vi "Calibrate.vi"() -> ()   [LabVIEW 2017]
panel:
  in  "Make New Calibration Setup":bool
  in  "Quit Calibration":bool
  in  "Load R.M.":bool
  in  "Load n":bool
  in  "Load S.F.":bool
  in  "Load P.M.":bool
  in  "Load Axial":bool
  in  "Load N.B.":bool
  out "Calibration Complete":bool
  out "Rolling Moment":bool
  out "n":bool
  out "S.F.":bool
  out "P.M.":bool
  out "Axial":bool
  out "Normal Beam":bool
  out "Current Calibration File Path":path
  in  "Load":bool
  in  "Use Old Calibration File Path":path
  # "Calibration Status"
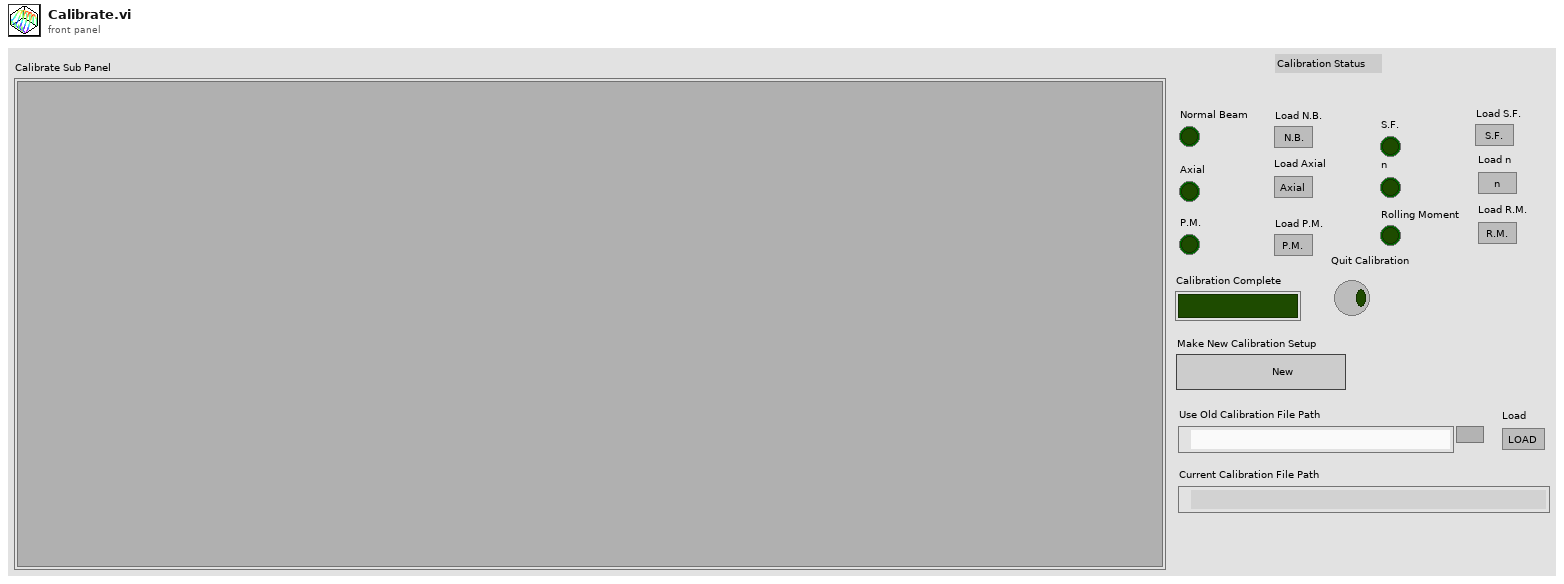
[diagram p1: front panel]
types:
  T1 = enum16{"open", "replace", "create", "open or create", "replace or create", "replace or create with confirmation"}
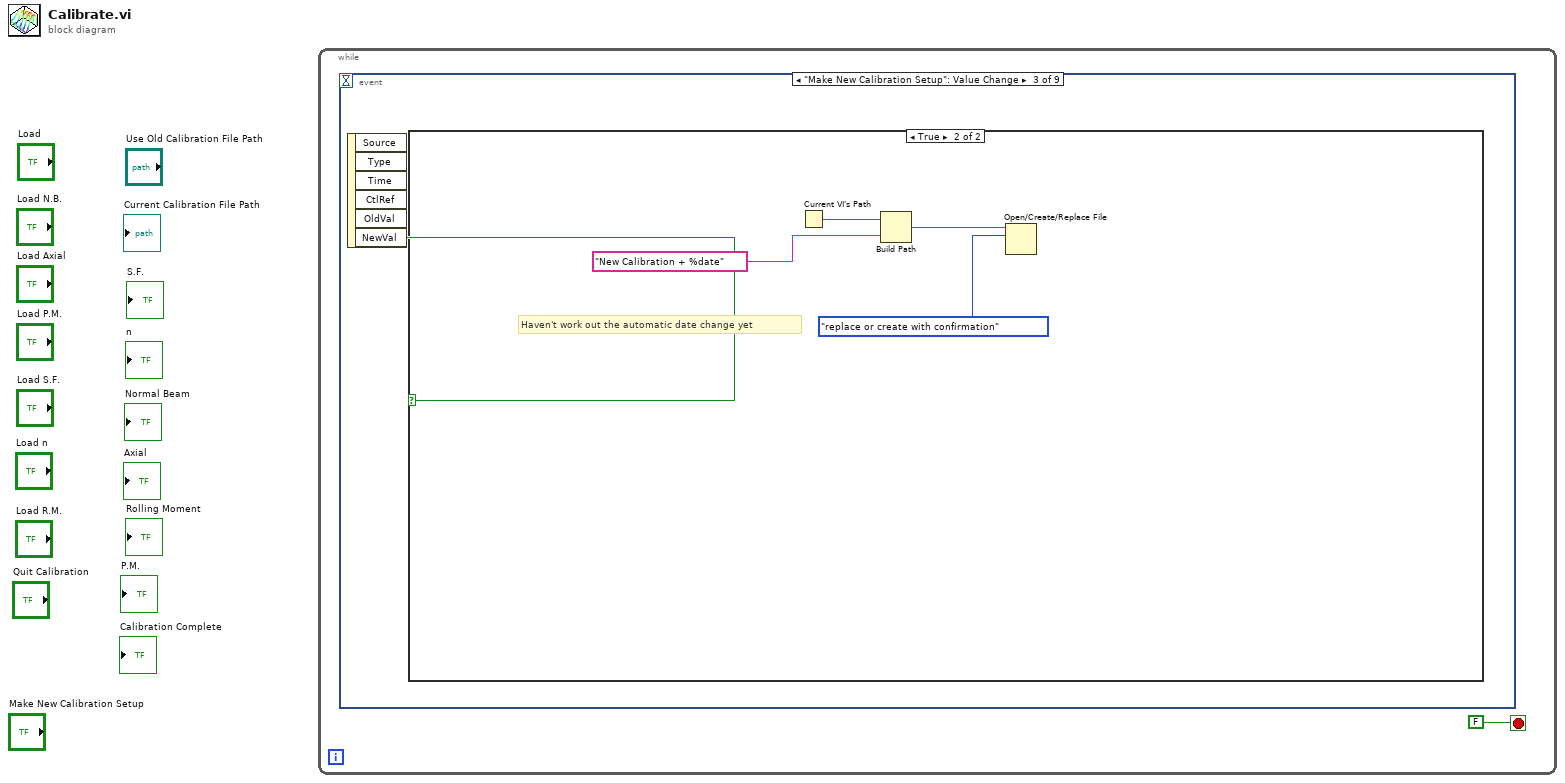
[diagram p0: block diagram]
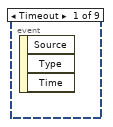
[diagram p2: hidden frame]
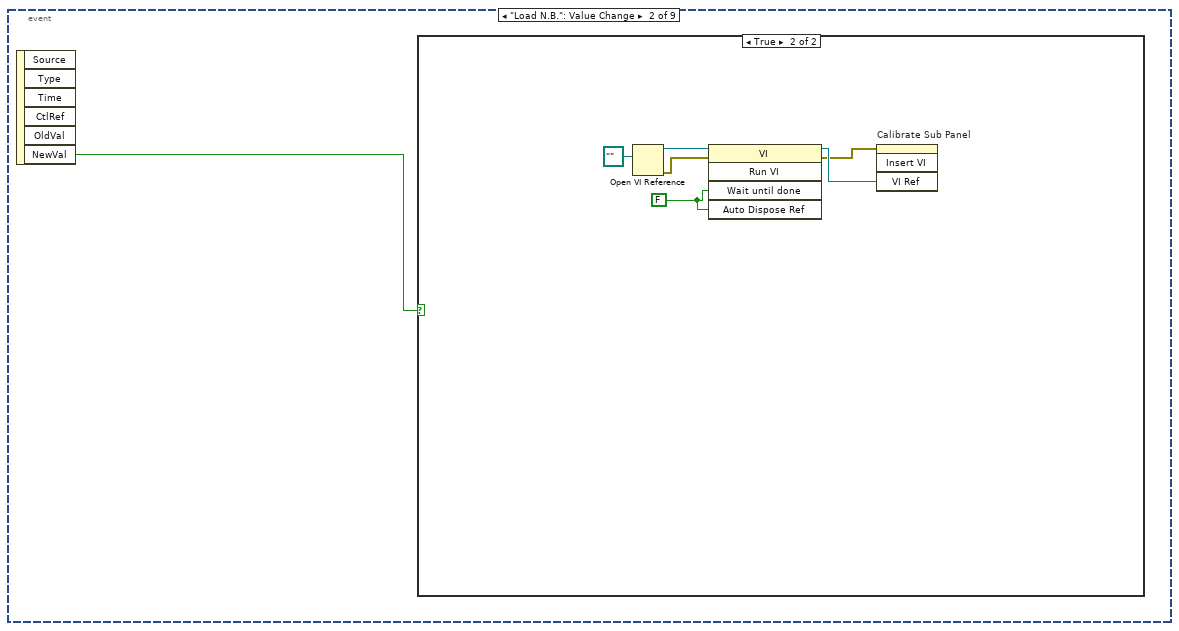
[diagram p3: hidden frame]
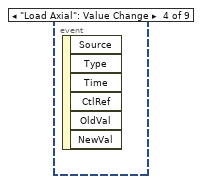
[diagram p6: hidden frame]
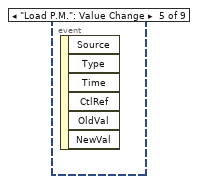
[diagram p7: hidden frame]
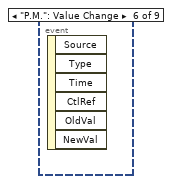
[diagram p8: hidden frame]
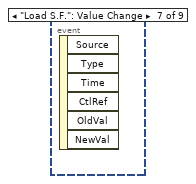
[diagram p9: hidden frame]
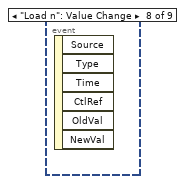
[diagram p10: hidden frame]
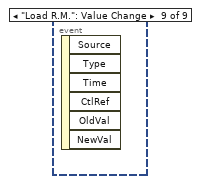
[diagram p11: hidden frame]
diagram:
  n1 = while {
    stop <- FALSE stop-if-true
    n2 = event shown="[2] \"Make New Calibration Setup\": Value Change" {
      selector: _ -> [_ _ _ _ _ _ _ _ _]
      dyn-events: _ -> [_ _ _ _ _ _ _ _ _]
      timeout: _ -> [_ _ _ _ _ _ _ _ _]
      event Timeout {
        n3 = event-data() -> ()  [unwired: 1 in, 3 out]
      }
      event "Load N.B.": Value Change {
        n4 = event-data() -> ("NewVal"=w2:bool)  [unwired: 1 in, 5 out]
        n5 = case shown="True" w2 {
          frame False {
          }
          frame True {
            w4 = FALSE ("Auto Dispose Reference")
            n6 = Open VI Reference(vi path=path "") -> (vi reference=w8:refnum<vi>, error out=w7:errorcluster)  [unwired: 5 in]
            n7 = invoke class="VI" method="Run VI"(reference=w8, error in=w7, "Wait until done"=w4, "Auto Dispose Ref"=w4) -> (reference out=w6:refnum<vi>, error out=w5:errorcluster)  [unwired: 1 in, 3 out]
            n8 = invoke on="Calibrate Sub Panel" class="SubPnl" method="Insert VI"(error in=w5, "VI Ref"=w6) -> ()  [unwired: 2 in, 4 out]
          }
        }
      }
      event "Make New Calibration Setup": Value Change {
        n9 = event-data() -> ("NewVal"=w9:bool)  [unwired: 1 in, 5 out]
        n10 = case shown="True" w9 {
          frame False {
          }
          frame True {
            # "Haven't work out the automatic date change yet"
            n11 = Current VI's Path() -> (path=w10:path)
            n12 = Build Path(base path=w10, name or relative path="New Calibration + %date") -> (appended path=w12:path)
            n13 = Open/Create/Replace File(file path (use dialog)=w12, operation (0:open)=T1."replace or create with confirmation") -> ()  [unwired: 4 in, 3 out]
          }
        }
      }
      event "Load Axial": Value Change {
        n14 = event-data() -> ()  [unwired: 1 in, 6 out]
      }
      event "Load P.M.": Value Change {
        n15 = event-data() -> ()  [unwired: 1 in, 6 out]
      }
      event "P.M.": Value Change {
        n16 = event-data() -> ()  [unwired: 1 in, 6 out]
      }
      event "Load S.F.": Value Change {
        n17 = event-data() -> ()  [unwired: 1 in, 6 out]
      }
      event "Load n": Value Change {
        n18 = event-data() -> ()  [unwired: 1 in, 6 out]
      }
      event "Load R.M.": Value Change {
        n19 = event-data() -> ()  [unwired: 1 in, 6 out]
      }
    }
  }
